vi "Log_create_logFile_pkcl.vi"(8 "errin":errorcluster caption="entrée d'erreur (pas d'erreur)", 10 "toute l'expression":string, 11 "Application Directory":path) -> (0 "sortie d'erreur":errorcluster, 1 "chemin complet":path, 3 "Fichier à flux d'octets en sortie":refnum<file>)   [LabVIEW 2020]
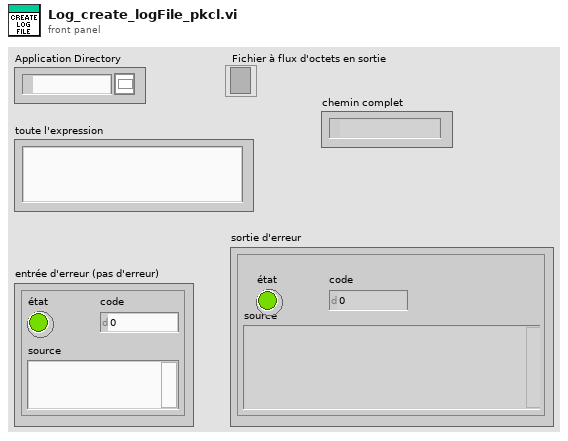
[diagram p1: front panel]
types:
  T1 = enum16{"open", "replace", "create", "open or create", "replace or create", "replace or create with confirmation"}
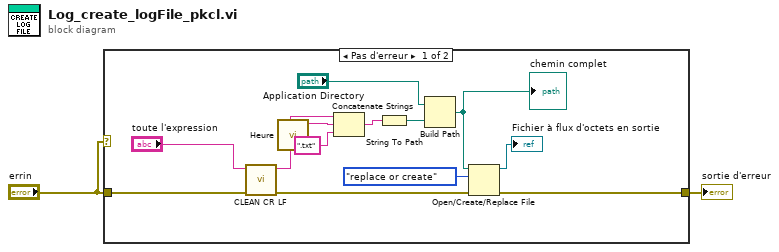
[diagram p0: block diagram]
diagram:
  n1 = case shown="Pas d'erreur" "errin" {
    tunnel: [w15 w16] -> w2
    tunnel: "errin" -> [w6 w16]
    frame No Error {
      n2 = call "CLEAN CR LF.vi"("errin"=w6, "in"="toute l'expression") -> ("errout"=w5:errorcluster, "out"=w3:string)  [unwired: 8 in]
      n3 = call "Heure.vi"() -> ("chaîne concaténée"=w13:string)  [unwired: 11 in]
      n4 = Concatenate Strings(w3, w13, ".txt" ("chaîne")) -> (w11:string)
      n5 = String To Path(string=w11) -> (path=w8:path)
      n6 = Build Path(base path="Application Directory", name or relative path=w8) -> (appended path=w10:path)
      "chemin complet" <- w10
      n7 = Open/Create/Replace File(file path (use dialog)=w10, error in=w5, operation (0:open)=T1."replace or create" ("opération (0 : open)")) -> (refnum out=→"Fichier à flux d'octets en sortie":refnum<file>, error out=w15:errorcluster)  [unwired: 3 in, 1 out]
    }
    frame Error {
    }
  }
  "sortie d'erreur" <- w2
